vi "Read Inputs (SubVI).vi"(8 "error in (no error)":errorcluster, 10 "Ports Ref In":bool[](array[boolean]), 11 "VISA Refnum in":refnum<visa-resource-name>) -> (0 "error out":errorcluster, 2 "Ports Ref Out":bool[](array[boolean]), 3 "VISA Refnum out":refnum<visa-resource-name>, 4 "LS":u32, 6 "Btn":u32)   [LabVIEW 2019]
doc: "En este VI se lleva a cabo la adquisición de datos de los sensores y de los pulsadores, conectados al PIC."
uses:
  <vilib>/Gustavo Trejo/PIC Serial Toolkit/Controls/Pin Number.ctl
panel:
  # "Entrada de datos:"
  # "Salida de datos:"
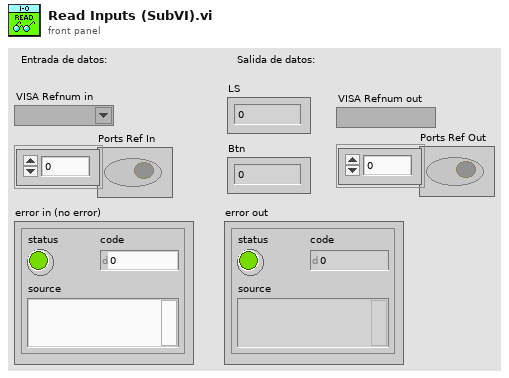
[diagram p1: front panel]
types:
  T1 = typedef "Pin Number.ctl" = enum16{"A0/AN0", "A1/AN1", "A2/AN2", "A3/AN3", "A4", "A5/AN4", "A6", "A7", "B0/AN12", "B1/AN10", "B2/AN8", "B3/AN9", "B4/AN11", "B5/AN13", "B6", "B7", "C0", "C1/PWM2", "C2/PWM1", "C3", "C4", "C5", "D0", "D1", "D2", "D3", "D4", "D5", "D6", "D7", "E0/AN5", "E1/AN6", "E2/AN7"}
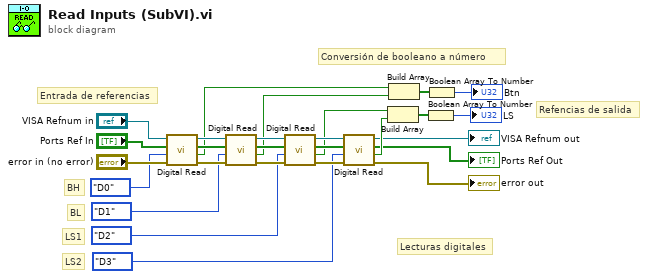
[diagram p0: block diagram]
diagram:
  # "Lecturas digitales"
  # "Entrada de referencias"
  # "Refencias de salida"
  # "Conversión de booleano a número"
  # "LS2"
  # "LS1"
  # "BL"
  # "BH"
  n1 = call <vilib>:"Digital Read.vi"("error in (no error)"="error in (no error)", "Pin Number"=Pin_Number."D0", "Ports Ref In"="Ports Ref In", "VISA Refnum in"="VISA Refnum in") -> ("error out"=w23:errorcluster, "Pin State Out"=w10:bool, "Ports Ref Out"=w22:bool[], "VISA Refnum out"=w21:refnum<visa-resource-name>)  [unwired: 4 in]
  n2 = call <vilib>:"Digital Read.vi"("error in (no error)"=w23, "Pin Number"=Pin_Number."D1", "Ports Ref In"=w22, "VISA Refnum in"=w21) -> ("error out"=w19:errorcluster, "Pin State Out"=w9:bool, "Ports Ref Out"=w18:bool[], "VISA Refnum out"=w17:refnum<visa-resource-name>)  [unwired: 4 in]
  n3 = call <vilib>:"Digital Read.vi"("error in (no error)"=w19, "Pin Number"=Pin_Number."D2", "Ports Ref In"=w18, "VISA Refnum in"=w17) -> ("error out"=w15:errorcluster, "Pin State Out"=w4:bool, "Ports Ref Out"=w14:bool[], "VISA Refnum out"=w13:refnum<visa-resource-name>)  [unwired: 4 in]
  n4 = call <vilib>:"Digital Read.vi"("error in (no error)"=w15, "Pin Number"=Pin_Number."D3", "Ports Ref In"=w14, "VISA Refnum in"=w13) -> ("error out"=→"error out":errorcluster, "Pin State Out"=w3:bool, "Ports Ref Out"=→"Ports Ref Out":bool[], "VISA Refnum out"=→"VISA Refnum out":refnum<visa-resource-name>)  [unwired: 4 in]
  n5 = Build Array(w4, w3) -> (w5:bool[])
  n6 = Build Array(w10, w9) -> (w8:bool[])
  n7 = Boolean Array To Number(Boolean array=w5) -> (number=→"LS":u32)
  n8 = Boolean Array To Number(Boolean array=w8) -> (number=→"Btn":u32)
